vi "SECoP_copy.vi"(8 "error in (no error)":errorcluster, 10 "SECoP_dataPtr in":T1 {"ptr64" format="%.0x"; "ptr32" format="%.0x"}, 11 "DLL path (in)":T2) -> (0 "error out":errorcluster, 2 "SECoP_dataPtr out":T1 {"ptr64" format="%.0x"; "ptr32" format="%.0x"}, 3 "DLL path (out)":T2)   [LabVIEW 2023, in "SECoP.lvlib"]
doc: "Call <b>\"SECoP_copy.vi\"</b> to make a deep copy of the data.\n\n<b>DLL path</b> input and output of cluster from \"SECoP-Initialize.vi\"\n<b>SECoP_dataPtr (in)</b> data to copy\n<b>SECoP_dataPtr (out)</b> fresh copy"
uses:
  SECoP.lvlib
  SECoP-libraries.ctl
  SECoP-data.ctl
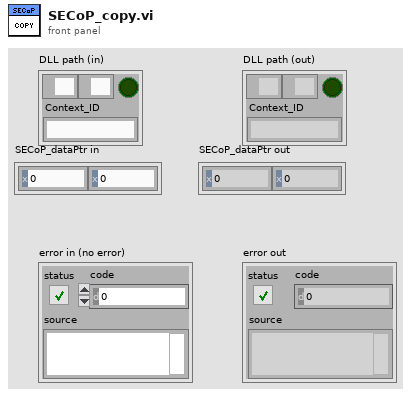
[diagram p1: front panel]
types:
  T1 = typedef "SECoP.lvlib/SECoP-data.ctl" = cluster{"ptr32":u32, "ptr64":u64}
  T2 = typedef "SECoP.lvlib/SECoP-libraries.ctl" = cluster{"serverDLL":path, "variantDLL":path, "cleanup_mode":bool, "Context_ID":string}
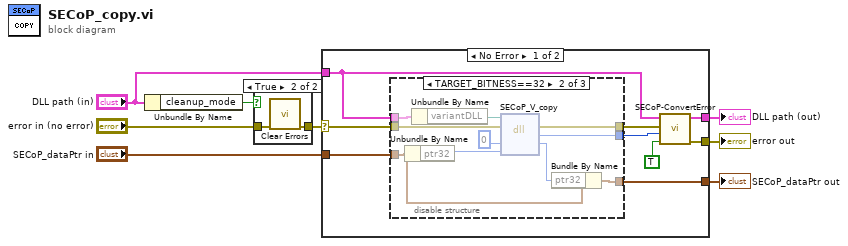
[diagram p0: block diagram]
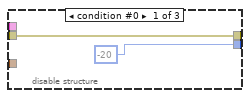
[diagram p3: hidden frame]
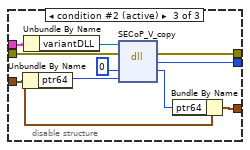
[diagram p4: hidden frame]
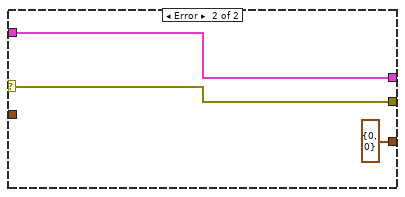
[diagram p5: hidden frame]
diagram:
  n1 = Unbundle By Name("DLL path (in)") -> ("cleanup_mode"=w6:bool)
  n2 = case shown="True" w6 {
    tunnel: "error in (no error)" -> [w9 w11]
    tunnel: [w9 w10] -> w4
    frame False {
    }
    frame True {
      n3 = call <vilib>:"Clear Errors.vi"("error in (no error)"=w11) -> ("error out"=w10:errorcluster)  [unwired: 5 in, 1 out]
    }
  }
  n4 = case shown="No Error" w4 {
    selector: w4 -> [w16 w44]
    tunnel: "DLL path (in)" -> [w12 w45]
    tunnel: [w19 w45] -> w8
    tunnel: [w20 w44] -> w7
    tunnel: "SECoP_dataPtr in" -> [w17 _]
    tunnel: [w13 T1 {"ptr32"=0, "ptr64"=0} ("SECoP_dataPtr in")] -> w2
    frame No Error {
      n5 = disable-structure shown="TARGET_BITNESS==32" {
        disable-tunnel: w17 -> [_ w27 w37]
        disable-tunnel: w16 -> [w21 w32 w42]
        disable-tunnel: w12 -> [_ w31 w41]
        disable-tunnel: [w21 w30 w40] -> w15
        disable-tunnel: [-20 w29 w39] -> w14
        disable-tunnel: [_ w26 w36] -> w13
        frame condition #0 {
        }
        frame condition #1 {
          n6 = Unbundle By Name(w27) -> ("ptr32"=w28:u32)
          n7 = Unbundle By Name(w31) -> ("variantDLL"=w23:path)
          n8 = dll-call lib="Z:/Praktische_Aufgaben/SECoP-LabVIEW2015/32bit/SECoP32.dll" fn="SECoP_V_copy"(path in=w23, error in=w32, "Dst"=u32 0 ("AdditionalBytes"), "Src"=w28) -> (error out=w30:errorcluster, "return type"=w29:i32, "Dst"=w25:u32)  [unwired: 2 in, 1 out]
          n9 = Bundle By Name(cluster=w27, "ptr32"=w25) -> (w26:T1)
        }
        frame condition #2 (active) {
          n10 = Unbundle By Name(w37) -> ("ptr64"=w38:u64)
          n11 = Unbundle By Name(w41) -> ("variantDLL"=w33:path)
          n12 = dll-call lib="Z:/Praktische_Aufgaben/SECoP-LabVIEW2015/32bit/SECoP32.dll" fn="SECoP_V_copy"(path in=w33, error in=w42, "Dst"=u64 0, "Src"=w38) -> (error out=w40:errorcluster, "return type"=w39:i32, "Dst"=w35:u64)  [unwired: 2 in, 1 out]
          n13 = Bundle By Name(cluster=w37, "ptr64"=w35) -> (w36:T1)
        }
      }
      n14 = call "SECoP-ConvertError.vi"("return is boolean"=TRUE, "return code"=w14, "error in (no error)"=w15, "DLL path (in)"=w12) -> ("error out"=w20:errorcluster, "DLL path (out)"=w19:T2)  [unwired: 6 in]
    }
    frame Error {
    }
  }
  "DLL path (out)" <- w8
  "error out" <- w7
  "SECoP_dataPtr out" <- w2
